vi "REC TRG.vi"(0 "System no.":i32=1 min=1 max=4 step=1, 2 "List of Data Recorder Trigger Configurations":T1[](array[typedef]), 5 "error in":errorcluster) -> (19 "error out":errorcluster)   [LabVIEW 2020]
doc: "REC TRG (Configure Data Recorder Trigger)\n\nDescription\nConfigures a data recorder for recording:\nSets the trigger that starts the recording. If necessary, REC TRG (p. 40) also configures the \nproperties of the trigger.\nA data recorder can only be configured when it is in the state \"CFG\", see the state diagram for \nthe data recorder (p. 110). The state of the data recorder can be queried with REC? STATE\n(p. 47). \n\nFormat\nREC TRG <RecorderID> <RecorderTrigger>[ <TriggerOption1>[ <TriggerOption2>]]\n\nArguments\n<RecorderID>\nData recorder, whose trigger is to be set; to be specified as alias (p. 94) \nThe available data recorders can be queried with USG? SYS (p. 80). \nPossible values: REC_1 to RECn, where n = number of data recorders in the controller\n<RecorderTrigger>\nTrigger for starting the recording\nThe available triggers can be queried with USG? PROP (p. 79). The response also indicates \nwhether additional arguments are required to configure the properties of the trigger; see the \n#Recorder Trigger block. \nPossible values:\nNOW = Default. Immediate trigger when sending REC START (p. 36); does not require any \nfurther configuration\nMOV = Triggers when the MOV command (p. 24) is sent; requires configuration using the \n<AxisID> and <Recurring> arguments\nOCV = Triggers when the OCV command (p. 26) is sent; requires configuration using the \n<AxisID> and <Recurring> arguments\nSMV = Triggers when the SMV command (p. 56) is sent; requires configuration using the \n<AxisID> and <Recurring> arguments\n<TriggerOption1>\nFirst argument for the configuration of the trigger\nSee the field <Option1> in block #Recorder Trigger. If the value is \"-\", the <TriggerOption1> and \n<TriggerOption2> arguments must be omitted in REC TRG.\nPossible values for <TriggerOption1> and <TriggerOption2>, see the response to USG? PROP:\n<AxisID>\nAn axis of the controller\nThe available axes can be queried with USG? SYS.\nPossible values: Alias of the axis (p. 94) \n<Recurring>\nShould repeated occurrences of the trigger start the recording again each time?\nPossible values:\n0 = \"Single\". Default. The first occurrence of the trigger starts the recording. Every other \noccurrence of the trigger has no effect.\n1 = \"Cyclic\". The first occurrence and every subsequent occurrence of the trigger starts a \nrecording.\n\nResponse\nnone\n\nExample\n>>rec? trg\n<<REC_1=NOW - - \n<<REC_2=NOW - -\n>>err?\n<<0 - (error 0 - \"No error\")\n>>rec trg rec_1 mov axis_1\n>>err?\n<<0 - (error 0 - \"No error\")\n>>rec? trg\n<<REC_1=MOV AXIS_1 0 \n<<REC_2=NOW - -\n>>rec trg rec_2 mov axis_2 1\n>>err?\n<<0 - (error 0 - \"No error\")\n>>rec? trg\n<<REC_1=MOV AXIS_1 0 \n<<REC_2=MOV AXIS_2 1\n\nNotes\nTo ensure that the set trigger is effective, the data recorder must be activated with REC START, \nwhich will set it to the state \"WAIT\" or \"RUN\".\nFor further details, see \"Data Recorder - GCS 3.0\" (p. 107). \n\nUser command level\nUSR"
uses:
  RecorderTriggerConfiguration.ctl
panel:
  # "REC TRG (Configure Data Recorder Trigger)\n\nConfigures a data recorder for recording:\nSets the trigger that starts the recording. If necessary, REC TRG also configures the properties of the trigger.\nA data recorder can only be configured when it is in the state \"CFG\", see the state diagram for the data recorder. The state of the data recorder can be queried with REC? STATE."
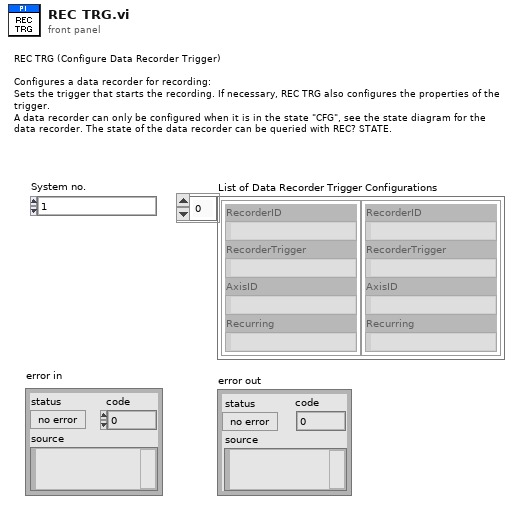
[diagram p1: front panel]
types:
  T1 = typedef "RecorderTriggerConfiguration.ctl" = cluster{"RecorderID":string, "RecorderTrigger":string, "AxisID":string, "Recurring":string}
  T2 = typedef "Syntax.ctl" = enum16{"GCS 1.0", "GCS 2.0", "GCS 3.0"}
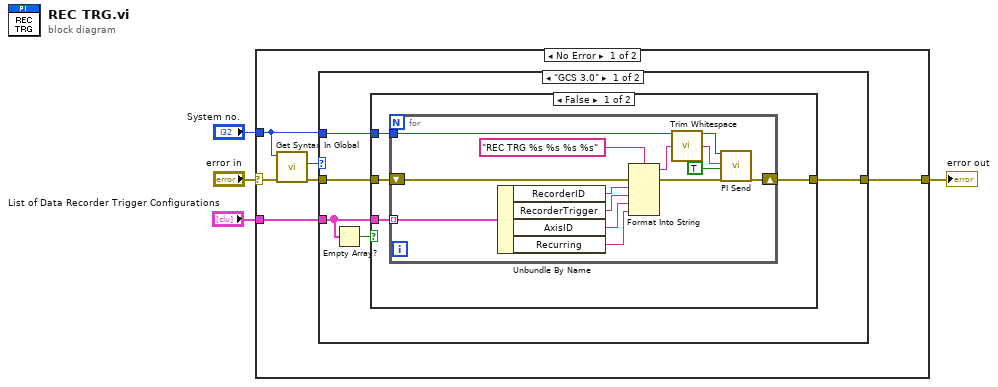
[diagram p0: block diagram]
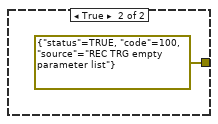
[diagram p2: hidden frame]
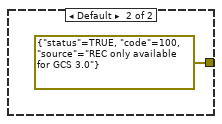
[diagram p3: hidden frame]
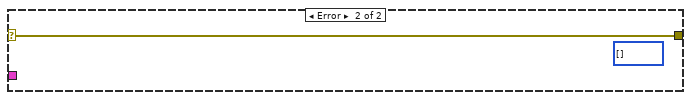
[diagram p4: hidden frame]
diagram:
  n1 = case shown="No Error" "error in" {
    selector: "error in" -> [w10 w35]
    tunnel: [w7 w35] -> w2
    tunnel: "System no." -> [w5 _]
    tunnel: "List of Data Recorder Trigger Configurations" -> [w6 _]
    frame No Error {
      n2 = call "Get Syntax In Global.vi"("error in"=w10, "System no."=w5) -> ("error out"=w8:errorcluster, "Syntax"=w9:T2)  [unwired: 8 in]
      n3 = case shown="\"GCS 3.0\"" w9 {
        tunnel: w8 -> [w15 _]
        tunnel: [w14 errorcluster {"status"=TRUE, "code"=100, "source"="REC only available for GCS 3.0"} ("error out")] -> w7
        tunnel: w5 -> [w13 _]
        tunnel: w6 -> [w11 _]
        frame "GCS 3.0" {
          n4 = Empty Array?(array=w11) -> (empty?=w12:bool)
          n5 = case shown="False" w12 {
            tunnel: w15 -> [w19 _]
            tunnel: [w18 errorcluster {"status"=TRUE, "code"=100, "source"="REC TRG empty parameter list"} ("error out")] -> w14
            tunnel: w13 -> [w17 _]
            tunnel: w11 -> [w16 _]
            frame False {
              n6 = for {
                shift-right: [w29] -> w18
                shift-left: w19 -> [w31]
                tunnel: w17 -> [w27]
                tunnel: w16 -> [w25] mode=indexing
                n7 = Unbundle By Name(w25) -> ("RecorderID"=w26:string, "RecorderTrigger"=w24:string, "AxisID"=w23:string, "Recurring"=w22:string)
                n8 = Format Into String(format string="REC TRG %s %s %s %s", error in=w31, w26, w24, w23, w22) -> (resulting string=w21:string, error out=w30:errorcluster)  [unwired: 1 in]
                n9 = call "Trim Whitespace.vi"("string"=w21) -> ("trimmed string"=w20:string)  [unwired: 1 in]
                n10 = call "PI Send.vi"("System no."=w27, "String to send"=w20, "Attach termination char.?"=TRUE, "error in"=w30) -> ("error out"=w29:errorcluster)  [unwired: 2 in, 13 out]
              }
            }
            frame True {
            }
          }
        }
        frame Default {
        }
      }
    }
    frame Error {
      (unwired) i32[] [] ("Number of recorded data points")
    }
  }
  "error out" <- w2
